vi "GCS3 Read Block.vi"(0 "GCS 3.0 Block to Parse":string, 2 "Expected GCS 3.0 Block Name":string, 3 "List of expected GCS 3.0 Block Entries":string[](array[string]), 5 "error in":errorcluster) -> (14 "List of extracted GCS 3.0 Block Entries":string[][](array[string]), 19 "error out":errorcluster)   [LabVIEW 2026]
uses:
  qLOG_State.ctl
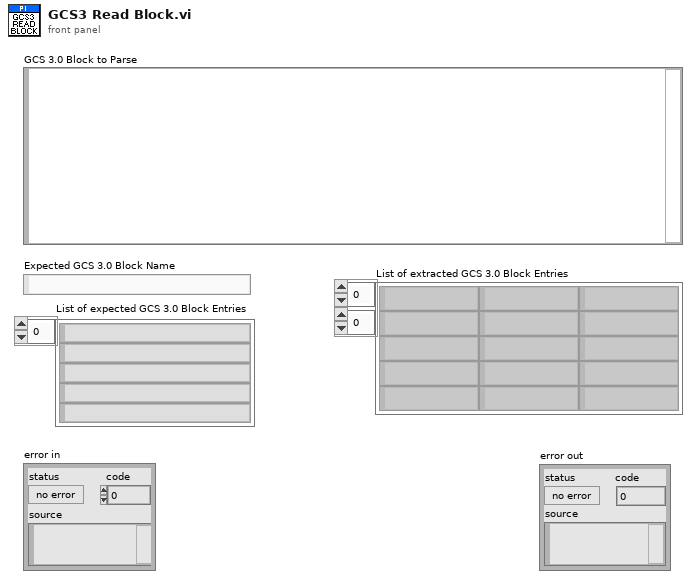
[diagram p1: front panel]
types:
  T1 = typedef "qLOG_State.ctl" = enum16{"Header", "Data"}
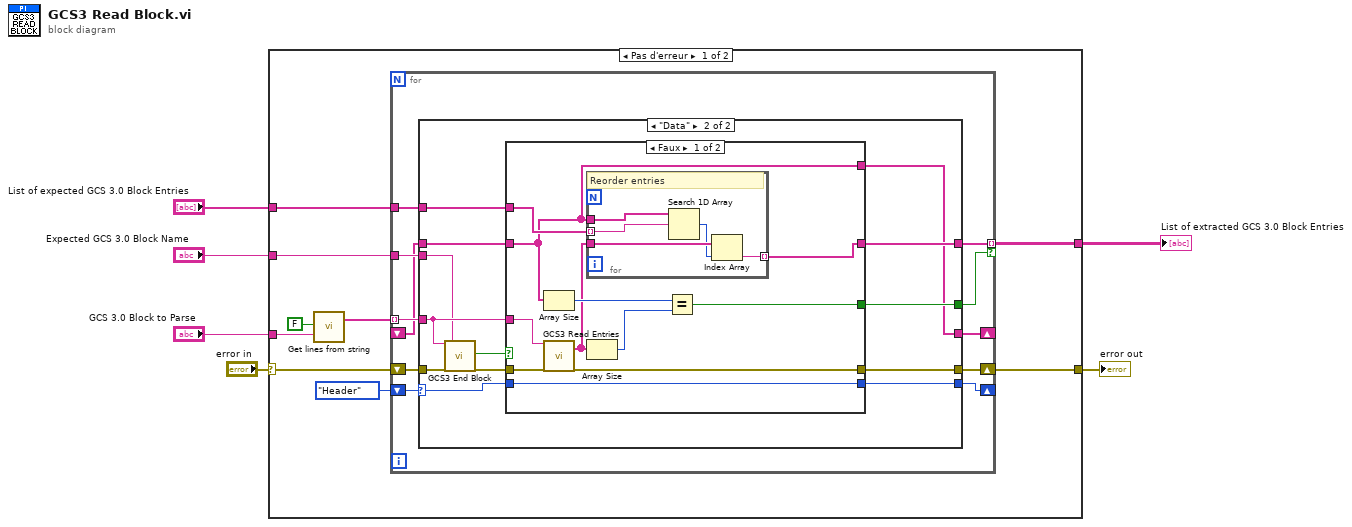
[diagram p0: block diagram]
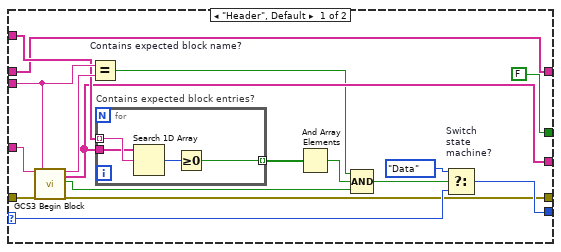
[diagram p2: hidden frame]
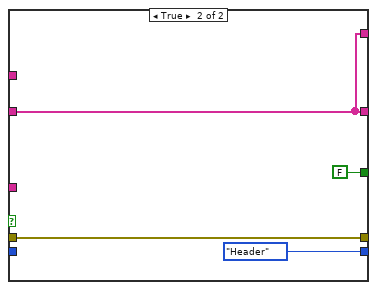
[diagram p3: hidden frame]
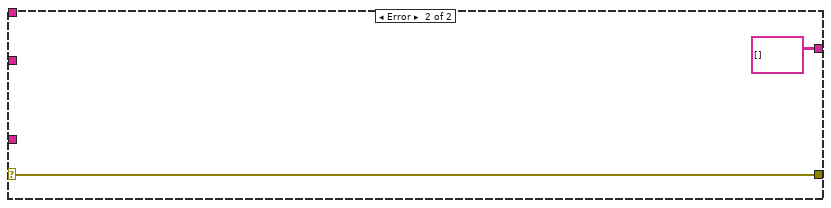
[diagram p4: hidden frame]
diagram:
  n1 = case shown="Pas d'erreur" "error in" {
    selector: "error in" -> [w11 w82]
    tunnel: [w10 w82] -> w5
    tunnel: "GCS 3.0 Block to Parse" -> [w14 _]
    tunnel: [w12 string[][] [] ("List of expected GCS 3.0 Block Entries")] -> w1
    tunnel: "List of expected GCS 3.0 Block Entries" -> [w7 _]
    tunnel: "Expected GCS 3.0 Block Name" -> [w8 _]
    frame No Error {
      n2 = call "Get lines from string.vi"("Cut spaces?"=FALSE, "Input string"=w14) -> ("Strings"=w13:string[])  [unwired: 16 in, 1 out]
      n3 = for {
        tunnel: w13 -> [w24] mode=indexing
        tunnel: [w20] -> w12 mode=indexing if=w21
        shift-right: [w22] -> _
        shift-left: qLOG_State."Header" ("LOG? State") -> [w23]
        shift-right: [w25] -> w10
        shift-left: w11 -> [w26]
        tunnel: w8 -> [w19]
        tunnel: w7 -> [w18]
        shift-right: [w17] -> _
        shift-left: _ -> [w16]
        n4 = case shown="\"Data\"" w23 {
          selector: w23 -> [w43 w56]
          tunnel: w26 -> [w41 w60]
          tunnel: [w42 w55] -> w22
          tunnel: [w40 w57] -> w25
          tunnel: w24 -> [w39 w58]
          tunnel: [w31 w54] -> w20
          tunnel: [FALSE w53] -> w21
          tunnel: w19 -> [w35 w52]
          tunnel: w18 -> [w34 w48]
          tunnel: [w32 w49] -> w17
          tunnel: w16 -> [w31 w50]
          frame "Header", Default {
            n5 = call "GCS3 Begin Block.vi"("Line to Parse"=w39, "error in"=w41, "Expected GCS 3.0 Block Name"=w35) -> ("GCS 3.0 Block Name"=w36:string, "Array of GCS 3.0 Block Entries"=w32:string[], "Is GCS 3.0 Block?"=w28:bool, "error out"=w40:errorcluster)  [unwired: 13 in]
            n6 = Equal? "Contains expected block name?"(x=w35, y=w36) -> (x = y?=w30:bool)
            n7 = for "Contains expected block entries?" {
              tunnel: w34 -> [w47] mode=indexing
              tunnel: w32 -> [w46]
              tunnel: [w44] -> w33 mode=indexing
              n8 = Search 1D Array(1D array=w46, element=w47) -> (index of element=w45:i32)  [unwired: 1 in]
              n9 = Greater Or Equal To 0?(x=w45) -> (x >= 0?=w44:bool)
            }
            n10 = And Array Elements(Boolean array=w33) -> (logical AND=w29:bool)
            n11 = Compound Arithmetic op=AND(w30, w29, w28) -> (w27:bool)
            n12 = Select "Switch\nstate\nmachine?"(t=qLOG_State."Data" ("LOG? State"), s=w27, f=w43) -> (s? t:f=w42:T1)
          }
          frame "Data" {
            n13 = call "GCS3 End Block.vi"("Line to Parse"=w58, "error in"=w60, "Expected GCS 3.0 Block Name"=w52) -> ("Is GCS 3.0 Block?"=w51:bool, "error out"=w59:errorcluster)  [unwired: 14 in, 1 out]
            n14 = case shown="Faux" w51 {
              tunnel: w59 -> [w70 w80]
              tunnel: w58 -> [w71 _]
              tunnel: [w69 w80] -> w57
              tunnel: w56 -> [w68 _]
              tunnel: [w68 qLOG_State."Header" ("LOG? State")] -> w55
              tunnel: w50 -> [w61 w77]
              tunnel: [w62 w77] -> w54
              tunnel: [w65 FALSE] -> w53
              tunnel: [w61 w77] -> w49
              tunnel: w48 -> [w64 _]
              frame False {
                n15 = Array Size(array=w61) -> (size(s)=w67:i32)
                n16 = call "GCS3 Read Entries.vi"("Line to Parse"=w71, "error in"=w70) -> ("Array of GCS 3.0 Block Entries"=w63:string[], "error out"=w69:errorcluster)  [unwired: 16 in]
                n17 = for {
                  tunnel: w64 -> [w76] mode=indexing
                  tunnel: w63 -> [w75]
                  tunnel: [w73] -> w62 mode=indexing
                  tunnel: w61 -> [w72]
                  # "Reorder entries"
                  n18 = Search 1D Array(1D array=w72, element=w76) -> (index of element=w74:i32)  [unwired: 1 in]
                  n19 = Index Array(array=w75, index=w74) -> (element=w73:string)
                }
                n20 = Array Size(array=w63) -> (size(s)=w66:i32)
                n21 = Equal?(x=w67, y=w66) -> (x = y?=w65:bool)
              }
              frame True {
              }
            }
          }
        }
      }
    }
    frame Error {
    }
  }
  "error out" <- w5
  "List of extracted GCS 3.0 Block Entries" <- w1
